vi "GaGe_ChannelConfig.vi"(3 "Channel (0)":u32 step=1, 4 "V scale":T2 {"Coupling" items=["DC 1 MOhm", "AC 1 MOhm", "DC 50 Ohm", "AC 50 OHM"]; "Offset" format="%.2f"}, 5 "Handle Cluster":T1) -> (2 "Handle Cluster Out":T1)   [LabVIEW 2022 SP3]
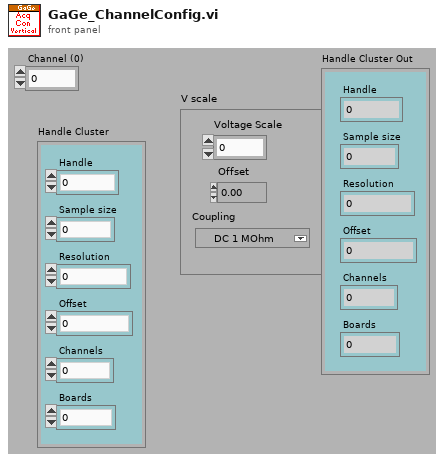
[diagram p1: front panel]
types:
  T1 = cluster{"Handle":u32, "Sample size":u32, "Resolution":i32, "Offset":i32, "Channels":u32, "Boards":u32}
  T2 = cluster{"Voltage Scale":dbl, "Offset":dbl, "Coupling":u16}
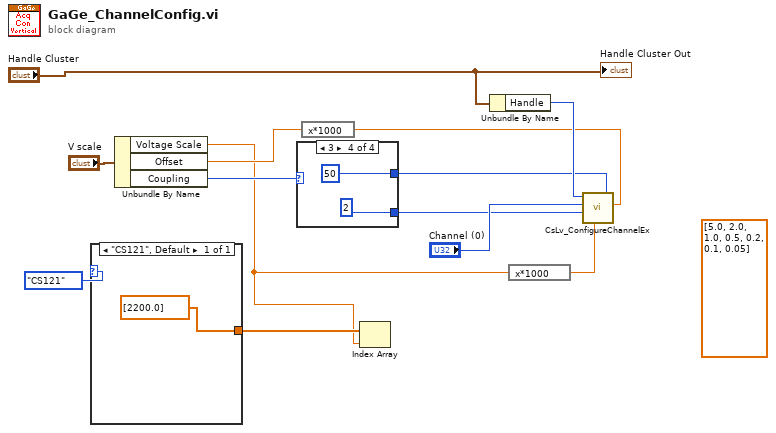
[diagram p0: block diagram]
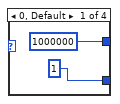
[diagram p2: hidden frame]
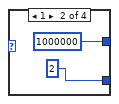
[diagram p3: hidden frame]
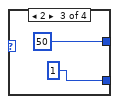
[diagram p4: hidden frame]
diagram:
  (unwired) dbl[] [5.0, 2.0, 1.0, 0.5, 0.2, 0.1, 0.05]
  n1 = case shown="\"CS121\", Default" enum16{"CS121", "DP 310"}."CS121" ("Enum") {
    tunnel: [dbl[] [2200.0]] -> w4
    frame "CS121", Default {
    }
  }
  n2 = Unbundle By Name("V scale") -> ("Voltage Scale"=w2:dbl, "Offset"=w7:dbl, "Coupling"=w10:u16)
  n3 = case shown="3" w10 {
    tunnel: [1000000 1000000 50 50] -> w9
    tunnel: [1 2 1 2] -> w8
    frame 0, Default {
    }
    frame 1 {
    }
    frame 2 {
    }
    frame 3 {
    }
  }
  n4 = expression code="x*1000"(w7) -> (w6:dbl)
  n5 = Index Array(array=w4, index=w2) -> ()  [unwired: 1 out]
  n6 = Unbundle By Name("Handle Cluster") -> ("Handle"=w12:u32)
  n7 = expression code="x*1000"(w2) -> (w1:dbl)
  n8 = call <userlib>:"CsLv_ConfigureChannelEx.vi"("DC Offset (0 mV)"=w6, "Impedance (1000000)"=w9, "Input range (2000 mV)"=w1, "Coupling (1)"=w8, "Channel (0)"="Channel (0)", "Handle"=w12) -> ()  [unwired: 3 in, 1 out]
  "Handle Cluster Out" <- "Handle Cluster"
